vi "Exception Nested Exception Throw.vi"(0 "details":string, 2 "Exception Nested Exception in":refnum<class "Exception Nested Exception.lvclass">, 11 "error in (no error)":errorcluster) -> (15 "error out":errorcluster)   [LabVIEW 2015, in "LV Exceptions v1.lvlib" / "Exception Nested Exception.lvclass"]
uses:
  Exception Nested Exception.lvclass
  Exception/Exception.lvclass/Exception.ctl
  Exception/Exception.lvclass
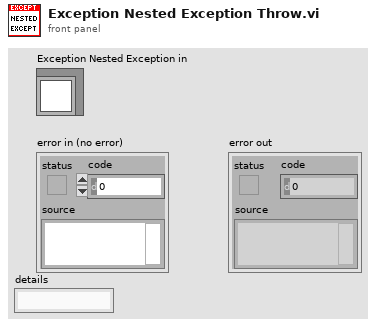
[diagram p1: front panel]
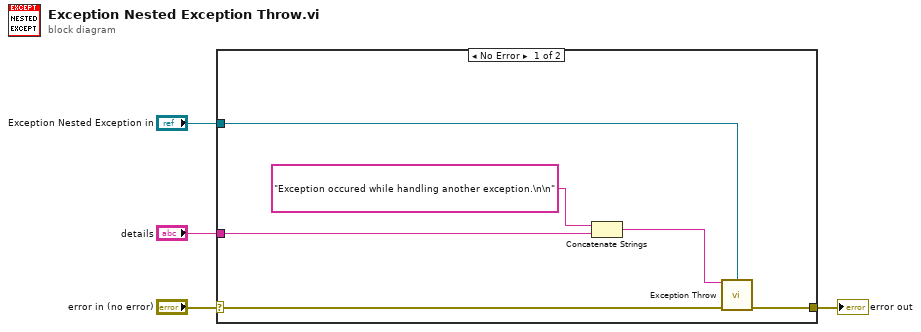
[diagram p0: block diagram]
diagram:
  n1 = case shown="No Error" "error in (no error)" {
    selector: "error in (no error)" -> [w10 w11]
    tunnel: [w9 w11] -> w3
    tunnel: "Exception Nested Exception in" -> [w8 _]
    tunnel: "details" -> [w5 _]
    frame No Error {
      n2 = Concatenate Strings("Exception occured while handling another exception.\n\n" ("message"), w5) -> (w6:string)
      n3 = call "Exception Throw.vi"("message"=w6, "Exception in"=w8, "error in (no error)"=w10) -> ("error out"=w9:errorcluster)  [unwired: 12 in]
    }
    frame Error {
    }
  }
  "error out" <- w3
